vi "Status Internal Plate Temperature Probe Alarm.vi"(8 "error in (no error)":errorcluster, 11 "heater_explorer in":refnum<class "heater_explorer.lvclass">) -> (0 "error out":errorcluster, 2 "Active?":bool, 3 "heater_explorer out":refnum<class "heater_explorer.lvclass">)   [LabVIEW 2020, in "polar_bear_plus_drivers.lvlib" / "heater_explorer.lvclass"]
doc: "Internal plate temperature probe does not exist."
uses:
  <instrlib>/RxnRover/Driver Polar Bear Plus/heater_explorer/heater_explorer.lvclass
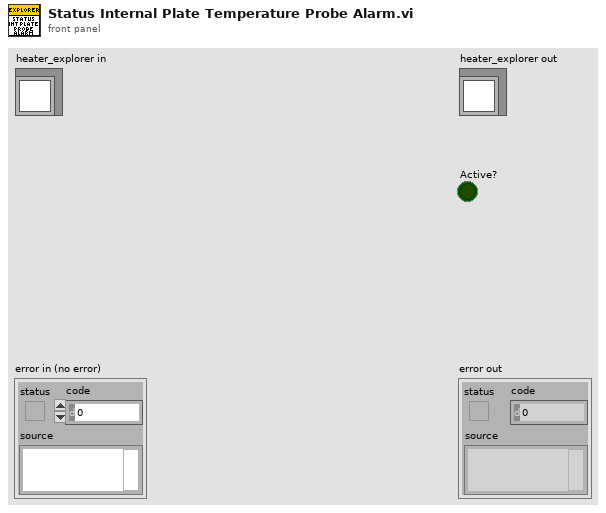
[diagram p1: front panel]
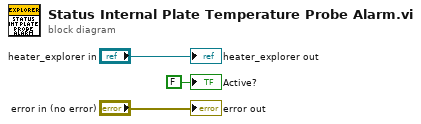
[diagram p0: block diagram]
diagram:
  "error out" <- "error in (no error)"
  "heater_explorer out" <- "heater_explorer in"
  "Active?" <- FALSE ("Active?")
